vi "Sound Input-Output.vi"() -> ()   [LabVIEW 2020]
doc: "This VI illustrates how to perform simultaneous sound IO, i.e., how to continuously play the sound acquired from a microphone. It requires the use of a microphone attached to the sound card. You can specify the IDs of the input and output devices, the frequency to sample at, and the buffer size for both devices. Higher frequencies have better quality, but demand more resources and are limited by the capabilities of your sound card. A large number of samples decreases the risk of glitches, but increases the delay between acquisition and playback."
uses:
  <vilib>/sound2/lvsound2.llb/Sampling Mode.ctl
  <vilib>/sound2/lvsound2.llb/Sound Data Format.ctl
  <vilib>/sound2/lvsound2.llb/Sound Output Write (DBL Single).vi
  <vilib>/sound2/lvsound2.llb/Sound Input Read (DBL).vi
  <vilib>/sound2/lvsound2.llb/Sound Output Write (DBL).vi
panel:
  out "CH2":waveform(dbl)(graph)
  out "CH1":waveform(dbl)(graph)
  in  "Stop":bool
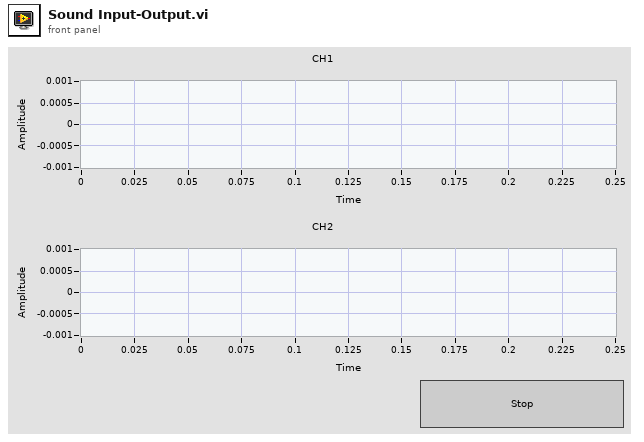
[diagram p1: front panel]
types:
  T1 = typedef "Sound Data Format.ctl" = cluster{"sample rate (S/s)":dbl, "number of channels":i32, "bits per sample":i32}
  T2 = typedef "Sampling Mode.ctl" = i32
  T3 = typedef "Sound Output Task ID.ctl" = u32
  T4 = typedef "Sound Input Task ID.ctl" = u32
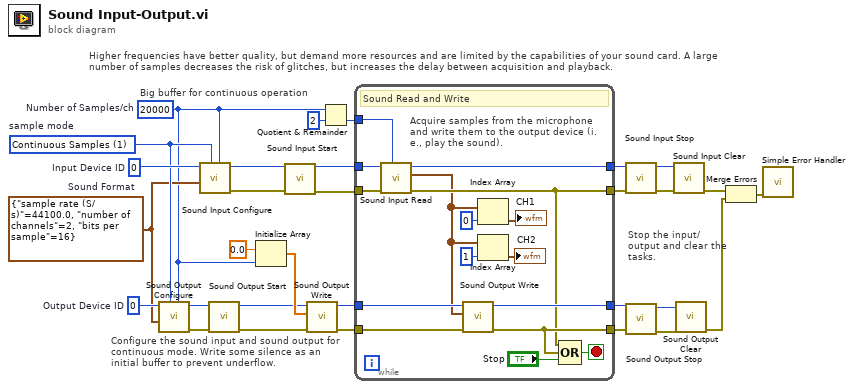
[diagram p0: block diagram]
diagram:
  w30 = u32 0  # Output Device ID
  w29 = u32 0  # Input Device ID
  w3 = 20000  # Number of Samples/ch
  w22 = T1 {"sample rate (S/s)"=44100.0, "number of channels"=2, "bits per sample"=16}  # Sound Format
  w26 = T2 1 items=["Finite Samples", "Continuous Samples"]  # sample mode
  # "Big buffer for continuous operation"
  # "Higher frequencies have better quality, but demand more resources and are limited by the capabilities of your sound card. A large number of samples decreases the risk of glitches, but increases the delay between acquisition and playback."
  # "Stop the input/output and clear the tasks."
  # "Configure the sound input and sound output for continuous mode. Write some silence as an initial buffer to prevent underflow."
  n1 = call <vilib>:"Sound Output Configure.vi"("number of samples/ch"=w3, "sample mode"=w26, "sound format"=w22, "device ID"=w30) -> ("error out"=w11:errorcluster, "task ID"=w10:T3)  [unwired: 6 in]
  n2 = call <vilib>:"Sound Input Configure.vi"("number of samples/ch"=w3, "sample mode"=w26, "sound format"=w22, "device ID"=w29) -> ("error out"=w7:errorcluster, "task ID"=w5:T4)  [unwired: 6 in]
  n3 = call <vilib>:"Sound Output Start.vi"("error in (no error)"=w11, "task ID"=w10) -> ("error out"=w9:errorcluster, "task ID out"=w8:T3)  [unwired: 8 in]
  n4 = Initialize Array(0.0 ("element"), w3) -> (w20:dbl[])
  n5 = call <vilib>:"Sound Input Start.vi"("error in (no error)"=w7, "task ID"=w5) -> ("error out"=w6:errorcluster, "task ID out"=w4:T4)  [unwired: 8 in]
  n6 = call-poly <vilib>:"Sound Output Write.vi"("error in (no error)"=w9, "data"=w20, "task ID"=w8) -> ("error out"=w25:errorcluster, "task ID out"=w24:T3)  [unwired: 7 in]
  n7 = Quotient & Remainder(x=w3, y=2) -> (floor(x/y)=w1:i32)  [unwired: 1 out]
  n8 = while {
    tunnel: w1 -> [w42]
    tunnel: w4 -> [w44]
    tunnel: [w41] -> w17
    tunnel: w24 -> [w45]
    tunnel: [w43] -> w15
    tunnel: w25 -> [w40]
    tunnel: [w37] -> w14
    tunnel: w6 -> [w46]
    tunnel: [w36] -> w19
    stop <- w39 stop-if-true
    # "Acquire samples from the microphone and write them to the output device (i.e., play the sound)."
    # "Sound Read and Write"
    n9 = call-poly <vilib>:"Sound Input Read.vi"("number of samples/ch"=w42, "error in (no error)"=w46, "task ID"=w44) -> ("error out"=w36:errorcluster, "data"=w31:waveform(dbl)[], "task ID out"=w41:T4)  [unwired: 6 in]
    n10 = call-poly <vilib>:"Sound Output Write.vi"("error in (no error)"=w40, "data"=w31, "task ID"=w45) -> ("error out"=w37:errorcluster, "task ID out"=w43:T3)  [unwired: 7 in]
    n11 = Index Array(array=w31, index=0) -> (element=→"CH1":waveform(dbl))
    n12 = Index Array(array=w31, index=1) -> (element=→"CH2":waveform(dbl))
    n13 = Compound Arithmetic op=OR(w36, w37, "Stop") -> (w39:bool)
  }
  n14 = call <vilib>:"Sound Input Stop.vi"("error in (no error)"=w19, "task ID"=w17) -> ("error out"=w18:errorcluster, "task ID out"=w16:T4)  [unwired: 8 in]
  n15 = call <vilib>:"Sound Output Stop.vi"("error in (no error)"=w14, "task ID"=w15) -> ("error out"=w12:errorcluster, "task ID out"=w13:T3)  [unwired: 8 in]
  n16 = call <vilib>:"Sound Input Clear.vi"("error in (no error)"=w18, "task ID"=w16) -> ("error out"=w27:errorcluster)  [unwired: 9 in]
  n17 = call <vilib>:"Sound Output Clear.vi"("error in (no error)"=w12, "task ID"=w13) -> ("error out"=w28:errorcluster)  [unwired: 9 in]
  n18 = Merge Errors(w27, w28) -> (w23:errorcluster)
  n19 = call <vilib>:"Simple Error Handler.vi"("error in (no error)"=w23) -> ()  [unwired: 4 in, 5 out]
